vi "SMC INIT.vi"   [LabVIEW 2010]
uses:
  TPS Global.vi
  <vilib>/Utility/config.llb/Read Key (String).vi
  SMC Global.vi
  <vilib>/Utility/config.llb/NI_LVConfig.lvlib
types:
  T1 = typedef "NI_LVConfig.lvlib/Config Data RefNum.ctl" = refnum<k1>
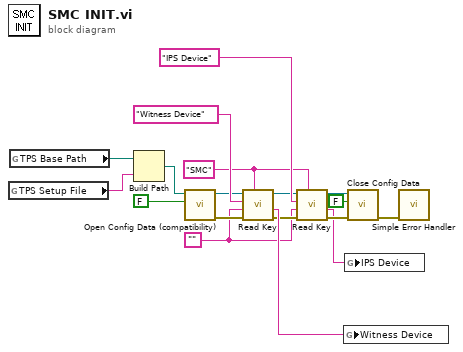
[diagram p0: block diagram]
diagram:
  w2 = ""
  w5 = "SMC" ("section")
  n1 = global read "TPS Global.vi" "TPS Setup File"() -> (w16:string)
  n2 = global read "TPS Global.vi" "TPS Base Path"() -> (w11:path)
  n3 = Build Path(base path=w11, name or relative path=w16) -> (appended path=w15:path)
  n4 = call <vilib>:"Open Config Data (compatibility).vi"("create file if necessary (T)"=FALSE ("create file if necessary? (T)"), "configuration file path"=w15) -> ("error out"=w13:errorcluster, "refnum"=w12:T1)  [unwired: 7 in, 1 out]
  n5 = call-poly <vilib>:"Read Key.vi"("section"=w5, "error in (no error)"=w13, "default value"=w2, "key"="Witness Device", "refnum"=w12) -> ("error out"=w4:errorcluster, "value"=w6:string, "refnum out"=w3:T1)  [unwired: 3 in, 1 out]
  n6 = call-poly <vilib>:"Read Key.vi"("section"=w5, "error in (no error)"=w4, "default value"=w2, "key"="IPS Device", "refnum"=w3) -> ("error out"=w10:errorcluster, "value"=w7:string, "refnum out"=w9:T1)  [unwired: 3 in, 1 out]
  n7 = global write "SMC Global.vi" "Witness Device"(w6) -> ()
  n8 = global write "SMC Global.vi" "IPS Device"(w7) -> ()
  n9 = call <vilib>:"Close Config Data.vi"("error in (no error)"=w10, "write file if changed (T)"=FALSE, "refnum"=w9) -> ("error out"=w18:errorcluster)  [unwired: 7 in, 1 out]
  n10 = call <vilib>:"Simple Error Handler.vi"("error in (no error)"=w18) -> ()  [unwired: 4 in, 5 out]
